vi "CalibrationLoadPrompt.vi"(11 "Root Path":path) -> (0 "cancel?":bool, 3 "selected path":path)   [LabVIEW 2024]
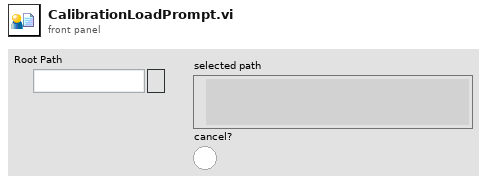
[diagram p1: front panel]
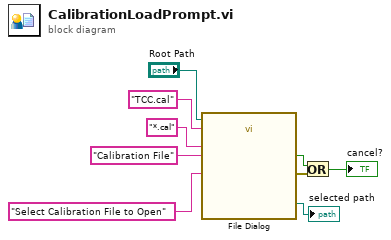
[diagram p0: block diagram]
diagram:
  n1 = call "File Dialog"("start path"="Root Path", "prompt"="Select Calibration File to Open", "default name"="TCC.cal", "pattern (all files)"="*.cal", "pattern label"="Calibration File") -> ("selected path"=→"selected path":path, "cancelled"=w8:bool, "error out"=w9:errorcluster)  [unwired: 7 in, 1 out]
  n2 = Or(x=w8, y=w9) -> (x .or. y?=→"cancel?":bool)
